vi "STepper_Calibrate.vi"() -> ()   [LabVIEW 2013]
panel:
  in  "Direction":bool=TRUE
  out "Numeric 2":i32
  in  "Numeric":i32
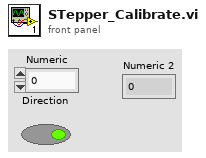
[diagram p1: front panel]
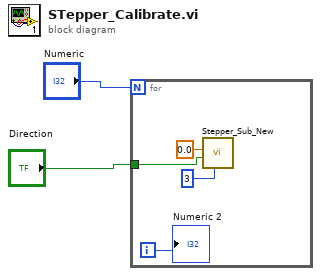
[diagram p0: block diagram]
diagram:
  n1 = for {
    N: "Numeric" -> [_]
    tunnel: "Direction" -> [w3]
    i -> [w4]
    n2 = call "Stepper_Sub_New.vi"("First Motor Pin"=u8 3, "Direction"=w3, "Velocity"=0.0) -> ()  [unwired: 7 in, 2 out]
    "Numeric 2" <- w4
  }
